vi "Get SMO Public API (This Level).vi"(8 "error in (no error)":errorcluster, 11 "Inst.RP100 in":refnum<class "Inst.RP100.lvclass">) -> (0 "error out":errorcluster, 2 "commands (this level)":string[](array[string]), 3 "Inst.RP100 out":refnum<class "Inst.RP100.lvclass">)   [LabVIEW 2019, in "Inst.RP100.lvclass"]
doc: "Override this VI to return a list of commands only supported by your Instrument"
uses:
  Inst.RP100.lvclass
  Typedefs/Inst.RP100.PublicCommands--Enum.ctl
  <userlib>/LevyLab/Instrument Framework/Instrument Types/Strain/Typedefs/Strain.Commands--Enum.ctl
  7d6b5044-c4df-427a-8517-ca438c78d292.vi
  3d10aecf-49ce-4c5f-be90-33055bcf045f.vi
  <vilib>/Utility/Data Type/Get Numeric Information.vi
  <userlib>/LevyLab/Instrument Framework/Instrument Types/Strain/Instrument.Strain.lvclass
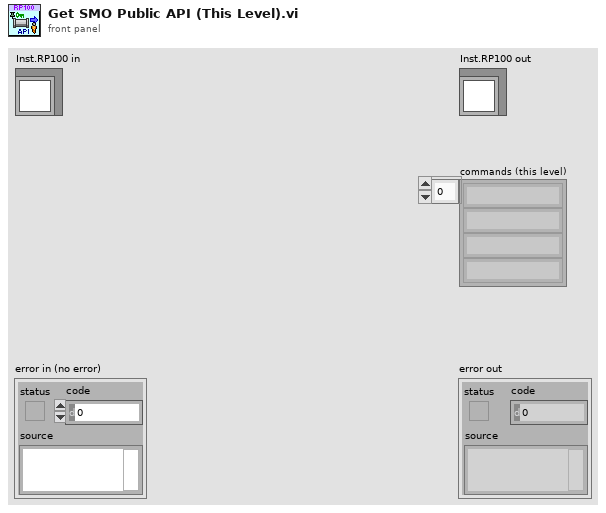
[diagram p1: front panel]
types:
  T1 = typedef "Instrument.Strain.lvclass/Strain.Commands--Enum.ctl" = enum16{"getStrain", "setStrain"}
  T2 = typedef "Inst.RP100.lvclass/Inst.RP100.PublicCommands--Enum.ctl" = enum16{"setState", "setLevel", "getLevel"}
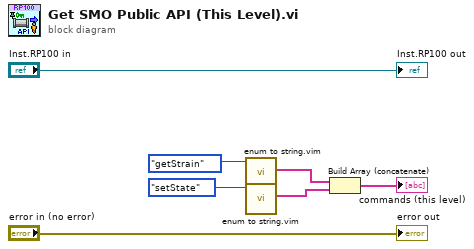
[diagram p0: block diagram]
diagram:
  n1 = call "enum to string.vim"("enum in"=Strain.Commands--Enum."getStrain" ("Command")) -> ("strings out"=w3:string[])  [unwired: 9 in, 1 out]
  n2 = call "enum to string.vim"("enum in"=Inst.RP100.PublicCommands--Enum."setState" ("Commands")) -> ("strings out"=w5:string[])  [unwired: 9 in, 1 out]
  n3 = Build Array (concatenate)(w3, w5) -> (→"commands (this level)":string[])
  "error out" <- "error in (no error)"
  "Inst.RP100 out" <- "Inst.RP100 in"
